vi "ReportTimeout.vi"(1 "Source":T1={"Subsystem Id"=3, "Node Id"=1, "Component Id"=1}, 2 "Destination":T1={"Subsystem Id"=90, "Node Id"=1, "Component Id"=1}, 3 "Sequence Number (16 bits)":u16=1) -> (8 "Encoded JAUS Message":string)   [LabVIEW 2009]
uses:
  Support Files/Address.ctl
panel:
  in  "Timeout":u8=10
  in  "Command Code":string="@\u0003"
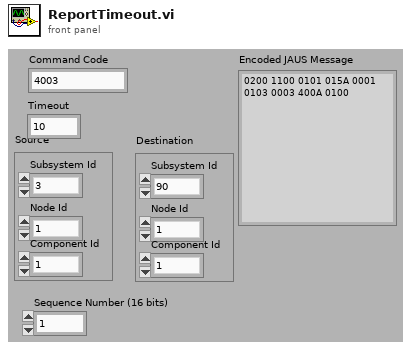
[diagram p1: front panel]
types:
  T1 = typedef "Address.ctl" = cluster{"Subsystem Id":u16, "Node Id":u8, "Component Id":u8}
  T2 = cluster{"unsigned byte array[0]":u8, "unsigned byte array[1]":u8}
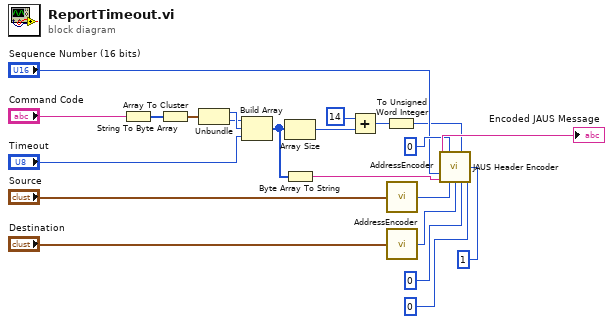
[diagram p0: block diagram]
diagram:
  n1 = String To Byte Array(string="Command Code") -> (unsigned byte array=w10:u8[])
  n2 = Array To Cluster(array=w10) -> (cluster=w9:T2)
  n3 = Unbundle(w9) -> ("unsigned byte array[0]"=w8:u8, "unsigned byte array[1]"=w7:u8)
  n4 = Build Array(w7, w8, "Timeout") -> (w13:u8[])
  n5 = Array Size(array=w13) -> (size(s)=w11:i32)
  n6 = Byte Array To String(unsigned byte array=w13) -> (string=w15:string)
  n7 = Add(x=14, y=w11) -> (x+y=w5:i32)
  n8 = To Unsigned Word Integer(number=w5) -> (unsigned 16bit integer=w4:u16)
  n9 = call "AddressEncoder.vi"("Address Cluster"="Source") -> ("Address"=w21:u32)
  n10 = call "AddressEncoder.vi"("Address Cluster"="Destination") -> ("Address"=w20:u32)
  n11 = call "JAUS Header Encoder.vi"("Message Type (0-5)"=u8 0, "Data Size (8-23)"=w4, "Priority(40-41)"=u8 1, "Sequence Number (16 bits)"="Sequence Number (16 bits)", "Payload"=w15, "Source ID (80-95)"=w21, "Destination ID (48-79)"=w20, "Data Flags (46-47)"=u8 0, "Ack/Nak (44-45)"=u8 0) -> ("Encoded JAUS Message"=→"Encoded JAUS Message":string)  [unwired: 6 in]
